vi "Constructor.vi"(6 "Precision":u8=6, 8 "error in":errorcluster, 9 "Value":dbl, 10 "Name":string, 11 "Decimal in":refnum<class "Decimal.lvclass">) -> (0 "error out":errorcluster, 3 "Decimal out":refnum<class "Decimal.lvclass">)   [LabVIEW 2021, in "ProligentXMLGenerator.lvlib" / "Decimal.lvclass"]
uses:
  Decimal.lvclass
  Decimal.lvclass/Decimal.ctl
  Attribute/Attribute.lvclass
  C:/Projects/proligent-xml-generator-labview/src/ProligentXMLGenerator/Base/Attribute/Attribute.lvclass
  C:/Projects/proligent-xml-generator-labview/src/ProligentXMLGenerator/Base/Decimal/Decimal.lvclass
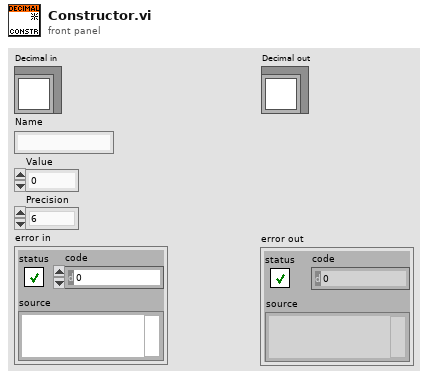
[diagram p1: front panel]
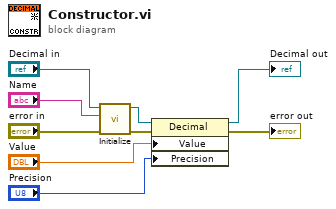
[diagram p0: block diagram]
diagram:
  n1 = call "Initialize.vi"("error in"="error in", "Name"="Name", "Attribute in"="Decimal in") -> ("error out"=w5:errorcluster, "Attribute out"=w4:refnum<class "Decimal.lvclass">)  [unwired: 7 in]
  n2 = property on="Property Node" class="Decimal"(reference=w4, error in=w5, "Value"="Value", "Precision"="Precision") -> (reference out=→"Decimal out":refnum<class "Decimal.lvclass">, error out=→"error out":errorcluster)
